vi "LabJackT4_Test.vi"() -> ()   [LabVIEW 2019]
uses:
  sub/enum_dev_id.ctl
  <vilib>/Analysis/baseanly.llb/Mean (DBL).vi
  <vilib>/Analysis/NI_AALBase.lvlib
panel:
  in  "clear_chart":bool caption="Clear charts to start"
  in  "dev_id":T1
  out "SN":i32
  in  "conn_type":T2(ring)
  out "avg_data":dbl[](array[numeric])
  out "Chart A":waveform(dbl)[](graph)
  out "Last Meas. Time":timestamp format="%<%Y-%m-%d %H:%M:%S>T"
  out "raw_data_size":i32[](array[numeric])
  in  "Read Rate (Hz)":dbl=1.0 format="%#_15g"
  in  "#Seconds on Graph":dbl=1.0 format="%.2f"
  out "Total Sample Rate (Hz)":dbl format="%.3f"
  out "ScansPerRead":i32
  out "ConnectionType Out":i32
  out "raw_data":dbl[][](array[numeric]) format="%.3f"
  out "Waveform Graph":dbl[][](graph)
  in  "Scan List":string[](array[string])=["AIN0", "AIN1", "AIN2", "AIN3", "AIN4", "AIN5", "AIN6", "AIN7", "AIN8", "AIN9", "AIN10", "AIN11"]
  out "iter":i32
  in  "Scan Rate (Hz)":dbl=5000.0 format="%.3f"
  in  "stop":bool
  out "Error Message":string
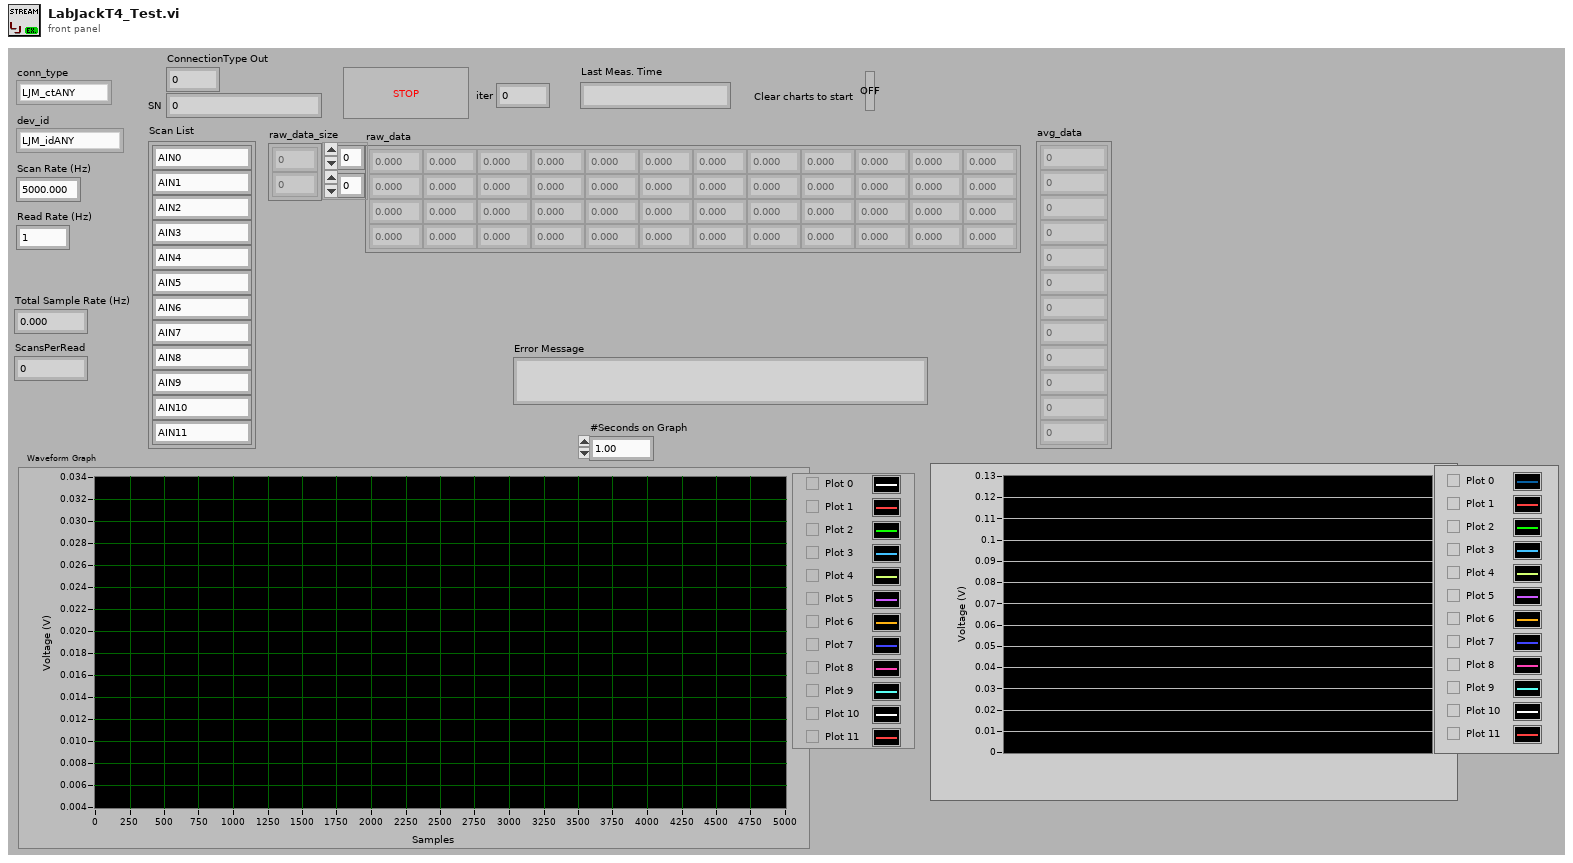
[diagram p1: front panel]
types:
  T1 = typedef "enum_dev_id.ctl" = enum16{"LJM_idANY", "192.168.24.185", "10.0.0.176", "440017305"}
  T2 = enum16{"LJM_ctANY", "LJM_ctUSB", "LJM_ctETHERNET"}
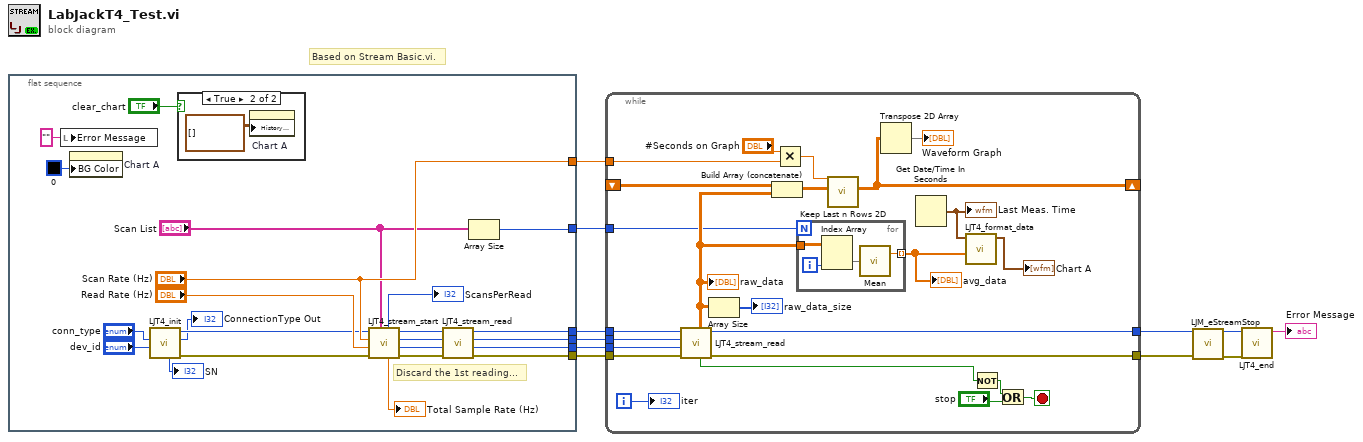
[diagram p0: block diagram]
diagram:
  # "Based on Stream Basic.vi."
  n1 = flat-sequence {
    tunnel: [w17] -> w11
    tunnel: [w16] -> w10
    tunnel: [w13] -> w4
    tunnel: [w14] -> w3
    tunnel: ["Scan Rate (Hz)"] -> w2
    tunnel: [w24] -> w1
    frame #0 {
      # "Discard the 1st reading..."
      n2 = local write "Error Message"("" ("Error Message")) -> ()
      n3 = property on="Chart A" class="WFChart (strict)"("BG Color"=u32 0 ("Plot Area:Colors:BG Color")) -> ()  [unwired: 2 in, 2 out]
      n4 = call "LJT4_init.vi"("dev_id"="dev_id", "conn_type"="conn_type") -> ("error out"=w30:errorcluster, "ConnectionType Out"=→"ConnectionType Out":i32, "Handle Out"=w27:i32, "SN"=→"SN":i32)  [unwired: 5 in, 1 out]
      n5 = case shown="True" "clear_chart" {
        frame False {
        }
        frame True {
          n6 = property on="Chart A" class="WFChart (strict)"("History Data"=waveform(dbl)[][] []) -> ()  [unwired: 2 in, 2 out]
        }
      }
      n7 = call "LJT4_stream_start.vi"("Scan List"="Scan List", "error in"=w30, "Read Rate (Hz)"="Read Rate (Hz)", "Scan Rate (Hz)"="Scan Rate (Hz)", "Handle in"=w27) -> ("error out"=w32:errorcluster, "NumReadAddresses"=w13:i32, "ScansPerRead Out"=w14:i32, "Handle out"=w15:i32, "Actual SampleRate"=→"Total Sample Rate (Hz)":dbl, "ScansPerRead"=→"ScansPerRead":i32)  [unwired: 1 in]
      n8 = call "LJT4_stream_read.vi"("error in"=w32, "NumReadAddresses"=w13, "ScansPerRead"=w14, "Handle in"=w15) -> ("error out"=w17:errorcluster, "Handle Out"=w16:i32)  [unwired: 4 in, 2 out]
      n9 = Array Size(array="Scan List") -> (size(s)=w24:i32)
    }
  }
  n10 = while {
    tunnel: [w52] -> w8
    tunnel: w10 -> [w53]
    tunnel: w4 -> [w50]
    tunnel: w3 -> [w49]
    shift-right: [w42] -> _
    shift-left: _ -> [w46]
    tunnel: w2 -> [w45]
    tunnel: w11 -> [w54]
    tunnel: [w51] -> w9
    tunnel: w1 -> [w38]
    i -> [w55]
    stop <- w56 stop-if-true
    n11 = call "LJT4_stream_read.vi"("error in"=w54, "NumReadAddresses"=w50, "ScansPerRead"=w49, "Handle in"=w53) -> ("error out"=w51:errorcluster, "Handle Out"=w52:i32, "status"=w41:bool, "data_out"=w39:dbl[][])  [unwired: 4 in]
    "raw_data" <- w39
    n12 = Array Size(array=w39) -> (size(s)=→"raw_data_size":i32[])
    n13 = Build Array (concatenate)(w46, w39) -> (w44:dbl[][])
    n14 = Multiply(x="#Seconds on Graph", y=w45) -> (x*y=w43:dbl)
    n15 = for {
      N: w38 -> [_]
      tunnel: w39 -> [w61]
      tunnel: [w58] -> w37 mode=indexing
      i -> [w60]
      n16 = Index Array(array=w61, index (col)=w60) -> (element=w59:dbl[])  [unwired: 1 in]
      n17 = call-poly <vilib>:"Mean.vi"("X"=w59) -> ("mean"=w58:dbl)  [unwired: 1 out]
    }
    "avg_data" <- w37
    n18 = call "Keep Last n Rows 2D.vi"("Array"=w44, "# Rows to Keep"=w43) -> ("Last n Rows"=w42:dbl[][])  [unwired: 9 in]
    n19 = Transpose 2D Array(2D array=w42) -> (transposed array=→"Waveform Graph":dbl[][])
    n20 = Get Date/Time In Seconds() -> (seconds since 1Jan1904=w36:timestamp)
    "Last Meas. Time" <- w36
    n21 = call "LJT4_format_data.vi"("value_array"=w37, "time"=w36) -> ("waveform_array_A"=→"Chart A":waveform(dbl)[])  [unwired: 9 in]
    n22 = Not(x=w41) -> (.not. x?=w34:bool)
    n23 = Or(x=w34, y="stop") -> (x .or. y?=w56:bool)
    "iter" <- w55
  }
  n24 = call "LJM_eStreamStop.vi"("Handle In"=w8, "error in"=w9) -> ("Handle Out"=w6:i32, "error out"=w7:errorcluster)  [unwired: 12 in]
  n25 = call "LJT4_end.vi"("error in (no error)"=w7, "Handle Out"=w6) -> ("String"=→"Error Message":string)  [unwired: 9 in]
